vi "Save File Create and Check For Summary File.vi"(7 "LV Program":T1=enum."DOE Stand", 8 "error in (no error)":errorcluster, 11 "File Paths In":T2={"General Setup Paths"={"Calibration File Path"=path "", "DOE Capacity Path"=path "", "Data Folder Path"=path "C:/", "RLT Backup Data Path"=path "", "Tool Base Path"=path "", "General Startup Config Path"=path "", "File Save Previous Run Path"=path "", "File Save Configuration Data Path"=path ""}, "Data File Paths"={"Data File Path"=path "", "Debug File Path"=path "", "Bus Log Path"=path "", "Current"=path "", "Summary"=path ""}, "New Summary Created"=FALSE, "Check Location Interval (Second)"=0}) -> (0 "error out":errorcluster, 3 "File Paths Out":T2={"General Setup Paths"={"Calibration File Path"=path "", "DOE Capacity Path"=path "", "Data Folder Path"=path "C:/", "RLT Backup Data Path"=path "", "Tool Base Path"=path "", "General Startup Config Path"=path "", "File Save Previous Run Path"=path "", "File Save Configuration Data Path"=path ""}, "Data File Paths"={"Data File Path"=path "", "Debug File Path"=path "", "Bus Log Path"=path "", "Current"=path "", "Summary"=path ""}, "New Summary Created"=FALSE, "Check Location Interval (Second)"=0})   [LabVIEW 2016, in "Save File.lvlib"]
uses:
  Save File.lvlib
  File Setup (Public)/Type Definition/Save File DOE File Path Control.ctl
  File Setup (Public)/Type Definition/Save File DOE Data Save Filepaths.ctl
  File Setup (Public)/Type Definition/Save File DOE LabView Program.ctl
  File Setup.lvlib
panel:
  in  "Summary":string="_Summary.csv"
  in  "Debug":string="_Debug Log.csv"
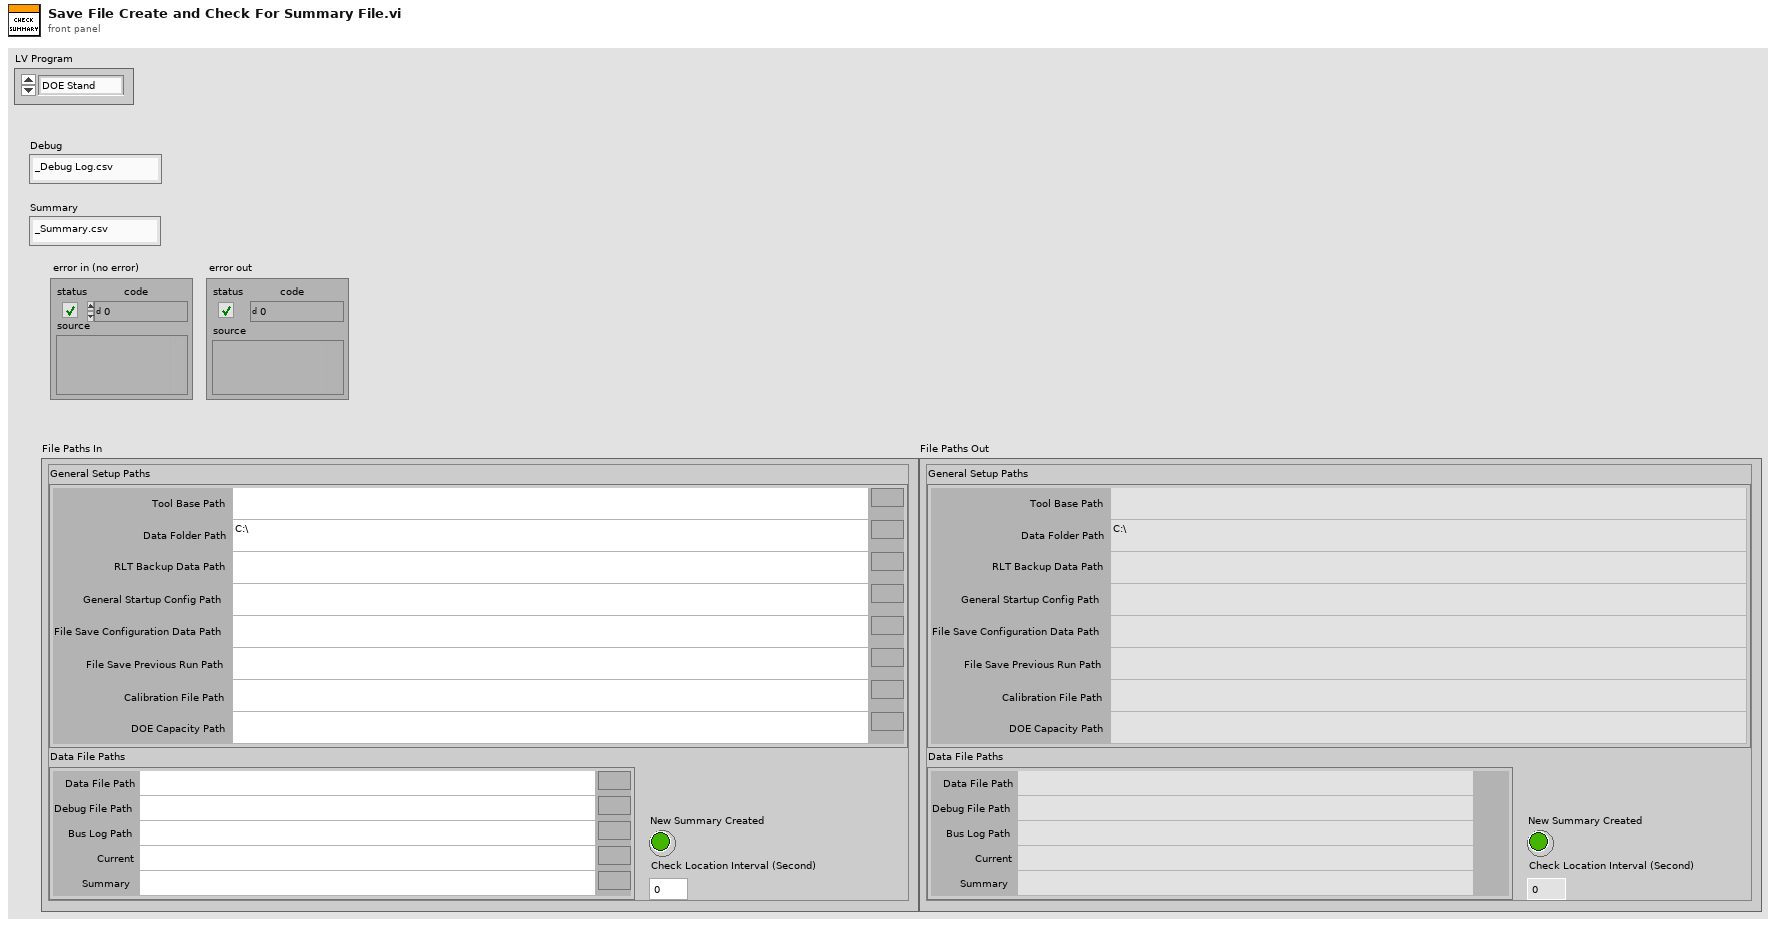
[diagram p1: front panel]
types:
  T1 = typedef "File Setup.lvlib/Save File DOE LabView Program.ctl" = enum16{"No Name Found", "DOE Stand", "Dishwasher Kitchen", "Portable Stand", "HEWH", "Dryer", "Dryer WILT", "HCC", "PRAT", "HEWH RLT", "Refrigeration"}
  T2 = typedef "File Setup.lvlib/Save File DOE File Path Control.ctl" = cluster{"General Setup Paths":cluster{"Calibration File Path":path, "DOE Capacity Path":path, "Data Folder Path":path, "RLT Backup Data Path":path, "Tool Base Path":path, "General Startup Config Path":path, "File Save Previous Run Path":path, "File Save Configuration Data Path":path}, "Data File Paths":T3, "New Summary Created":bool, "Check Location Interval (Second)":i32}
  T3 = typedef "File Setup.lvlib/Save File DOE Data Save Filepaths.ctl" = cluster{"Data File Path":path, "Debug File Path":path, "Bus Log Path":path, "Current":path, "Summary":path}
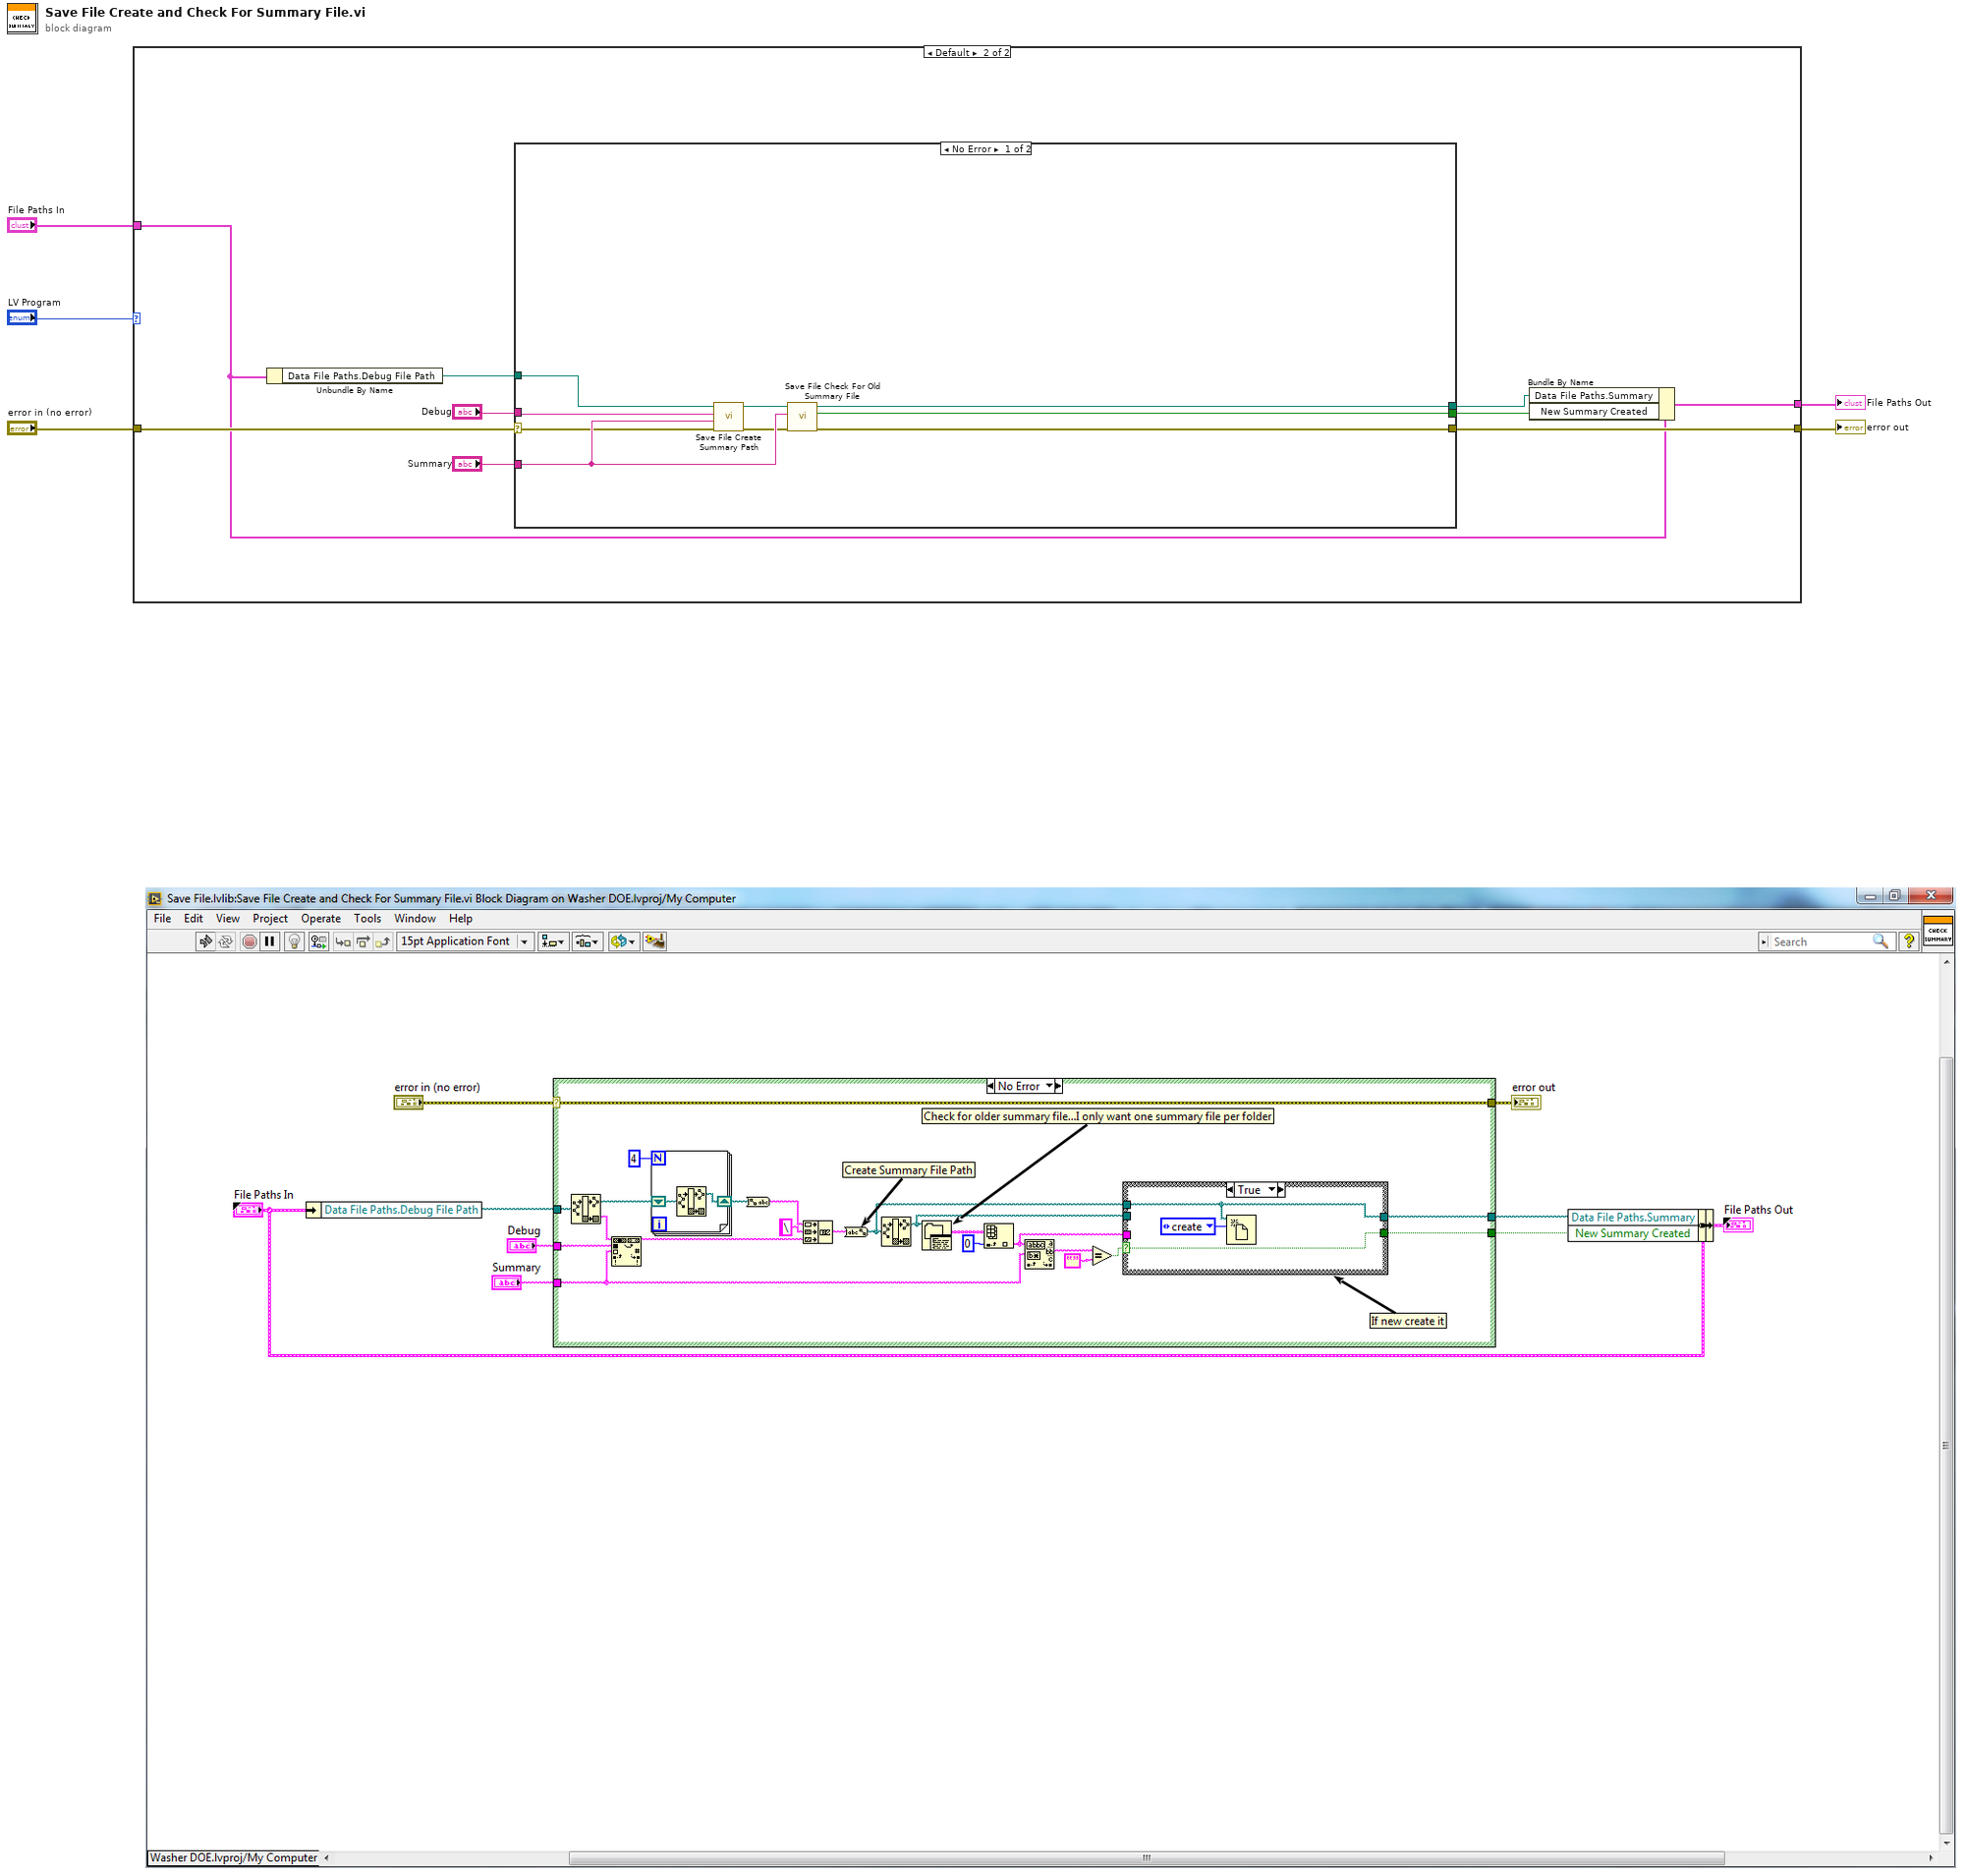
[diagram p0: block diagram]
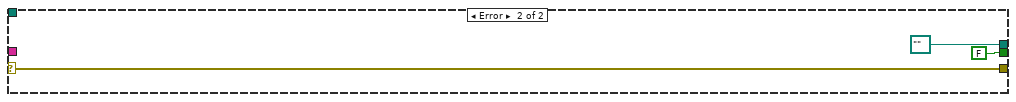
[diagram p3: hidden frame]
diagram:
  n1 = case shown="Default" "LV Program" {
    tunnel: "error in (no error)" -> [w7 w11]
    tunnel: [w7 w10] -> w3
    tunnel: "File Paths In" -> [w6 w9]
    tunnel: [w6 w8] -> w1
    frame "Refrigeration" {
    }
    frame Default {
      n2 = Unbundle By Name(w9) -> ("Data File Paths.Debug File Path"=w14:path)
      n3 = case shown="No Error" w11 {
        selector: w11 -> [w18 w28]
        tunnel: [w25 FALSE] -> w12
        tunnel: w14 -> [w24 _]
        tunnel: [w23 path ""] -> w13
        tunnel: "Summary" -> [w22 _]
        tunnel: "Debug" -> [w20 _]
        tunnel: [w17 w28] -> w10
        frame No Error {
          n4 = call "Save File Create Summary Path.vi"("Error In"=w18, "Summary"=w22, "Debug"=w20, "Debug File Path"=w24) -> ("Error Out"=w19:errorcluster, "Path"=w21:path)  [unwired: 6 in]
          n5 = call "Save File Check For Old Summary File.vi"("Error In"=w19, "Summary"=w22, "Path in"=w21) -> ("Error Out"=w17:errorcluster, "New Summary Created"=w25:bool, "Path out"=w23:path)  [unwired: 6 in]
        }
        frame Error {
        }
      }
      n6 = Bundle By Name(cluster=w9, "Data File Paths.Summary"=w13, "New Summary Created"=w12) -> (w8:T2)
    }
  }
  "error out" <- w3
  "File Paths Out" <- w1
